vi "Volt_to_board_0.vi"(8 "error in (no error)":errorcluster, 9 "values to write":u8[](array[numeric]) format="%02x", 10 "addresses":u32[](array[numeric]) format="%04x", 11 "board":refnum<visa-resource-name>="PXI4::5::INSTR") -> (0 "error out":errorcluster)   [LabVIEW 2015]
doc: "This VI writes the <b>values to write</b> to the <b>addresses</b> for the specified <b>board</b>."
uses:
  <vilib>/Instr/_visa.llb/VISA Register Access Address Space.ctl
panel:
  out "Boolean":bool
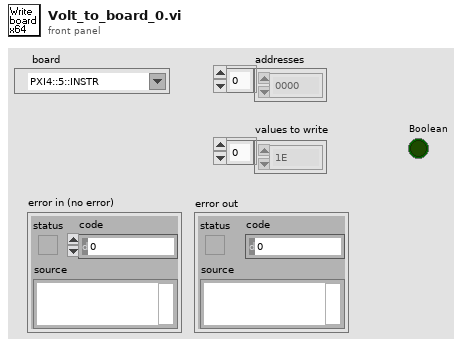
[diagram p1: front panel]
types:
  T1 = typedef "VISA Register Access Address Space.ctl" = u16
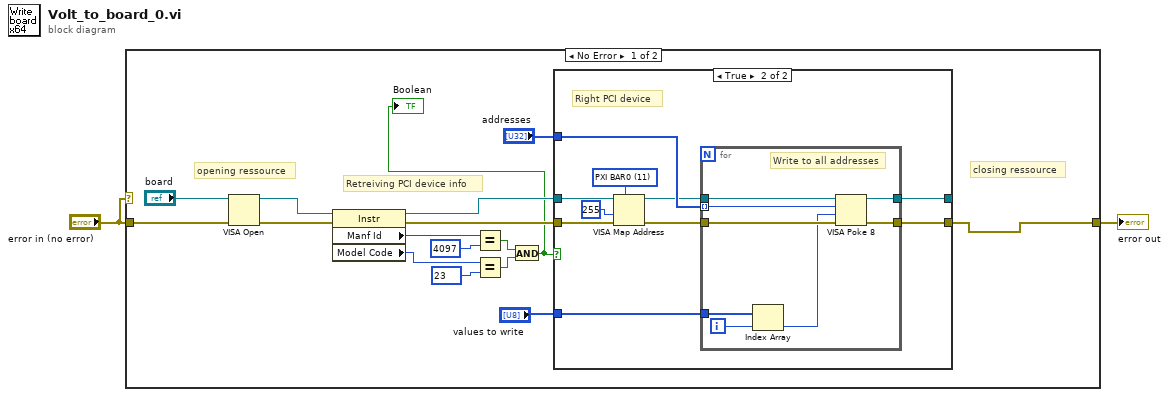
[diagram p0: block diagram]
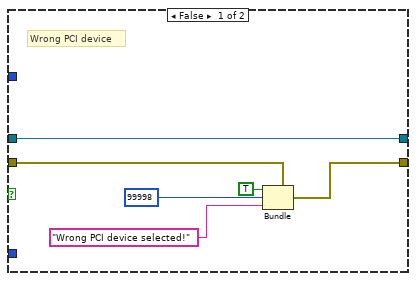
[diagram p2: hidden frame]
diagram:
  n1 = case shown="No Error" "error in (no error)" {
    tunnel: "error in (no error)" -> [w17 w43]
    tunnel: [w4 w43] -> w2
    frame No Error {
      # "closing ressource"
      # "opening ressource"
      # "Retreiving PCI device info"
      n2 = VISA Open(error in (no error)=w17, VISA resource name="board") -> (VISA resource name=w16:refnum<visa-resource-name>, error out=w15:errorcluster)  [unwired: 3 in]
      n3 = property class="Instr"(reference=w16, error in=w15) -> (reference out=w10:refnum<visa-resource-name>, error out=w7:errorcluster, "Manf Id"=w6:u16, "Model Code"=w5:u16)
      n4 = Equal?(x=w6, y=u16 4097) -> (x = y?=w12:bool)
      n5 = Equal?(x=w5, y=u16 23) -> (x = y?=w13:bool)
      n6 = And(x=w12, y=w13) -> (x .and. y?=w3:bool)
      "Boolean" <- w3
      n7 = case shown="True" w3 {
        tunnel: [w24 w34] -> _
        tunnel: w10 -> [w24 w30]
        tunnel: w7 -> [w20 w29]
        tunnel: [w19 w33] -> w4
        tunnel: "addresses" -> [_ w32]
        tunnel: "values to write" -> [_ w25]
        frame False {
          # "Wrong PCI device"
          n8 = Bundle(cluster=w20, "status"=TRUE, "code"=99998, "source"="Wrong PCI device selected!") -> (w19:errorcluster)
        }
        frame True {
          w27 = T1 11 items=["VXI/VME A16"=1, "VXI/VME A24"=2, "VXI/VME A32"=3, "VXI/VME A64"=4, "PXI Memory Allocations"=9, "PXI Configuration"=10, "PXI BAR0"=11, "PXI BAR1"=12, "PXI BAR2"=13, "PXI BAR3"=14, "PXI BAR4"=15, "PXI BAR5"=16] ("Address Space")
          # "Right PCI device"
          n9 = VISA Map Address(7:w27, 8:w29, 9:u32 255 ("map size (0)"), 11:w30) -> (0:w28:errorcluster, 3:w31:refnum<visa-resource-name>)  [unwired: 2 in]
          n10 = for {
            tunnel: w31 -> [w39]
            tunnel: [w42] -> w34
            tunnel: w28 -> [w41]
            tunnel: [w40] -> w33
            tunnel: w32 -> [w38] mode=indexing
            tunnel: w25 -> [w36]
            i -> [w35]
            # "Write to all addresses"
            n11 = Index Array(array=w36, index=w35) -> (element=w37:u8)
            n12 = VISA Poke 8(8:w41, 9:w37, 10:w38, 11:w39) -> (0:w40:errorcluster, 3:w42:refnum<visa-resource-name>)
          }
        }
      }
    }
    frame Error {
    }
  }
  "error out" <- w2
